vi "test Add Alias With Extra Empty Items.vi"(8 "error in (no error)":errorcluster, 11 "TestCase in":refnum<class "Routing and Faulting Aliases Unit Tests.lvclass">) -> (0 "error out":errorcluster, 3 "TestCase out":refnum<class "Routing and Faulting Aliases Unit Tests.lvclass">)   [LabVIEW 2019, in "Routing and Faulting Aliases Unit Tests.lvclass"]
uses:
  Routing and Faulting Aliases Unit Tests.lvclass
  System Explorer/Alias.ctl
  System Explorer/Endpoint.ctl
  Shared/Alias Endpoint.ctl
  Shared/Alias Mapping.ctl
  Routing and Faulting Aliases Unit Tests.lvclass/Routing and Faulting Aliases Unit Tests.ctl
  <vilib>/addons/_JKI Toolkits/VI Tester/TestCase.llb/TestCase.lvclass
  System Explorer/Routing and Faulting System Explorer.lvlib
  Scripting/Routing and Faulting Scripting.lvlib
  Shared/Routing and Faulting Shared.lvlib
  C:/Program Files (x86)/National Instruments/LabVIEW 2019/vi.lib/addons/_JKI Toolkits/VI Tester/TestCase.llb/TestCase.lvclass
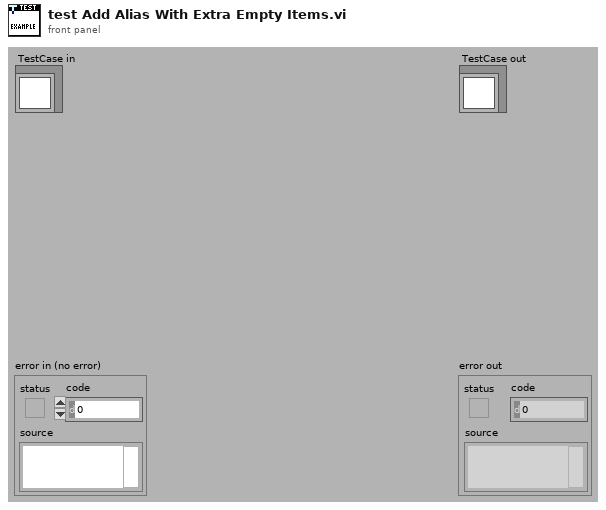
[diagram p1: front panel]
types:
  T1 = typedef "Routing and Faulting Shared.lvlib/Alias Mapping.ctl" = cluster{"Alias":string, "Endpoint":T2}
  T2 = typedef "Routing and Faulting Shared.lvlib/Alias Endpoint.ctl" = cluster{"Module Path":string, "Endpoint":string}
  T3 = typedef "Routing and Faulting System Explorer.lvlib/Endpoint.ctl" = string
  T4 = typedef "Routing and Faulting System Explorer.lvlib/Alias.ctl" = cluster{"Endpoint":T3, "Alias":string, "Remove":bool}
  T5 = typedef "Custom Device API.lvlib/Custom Device Item Ref.ctl" = u64
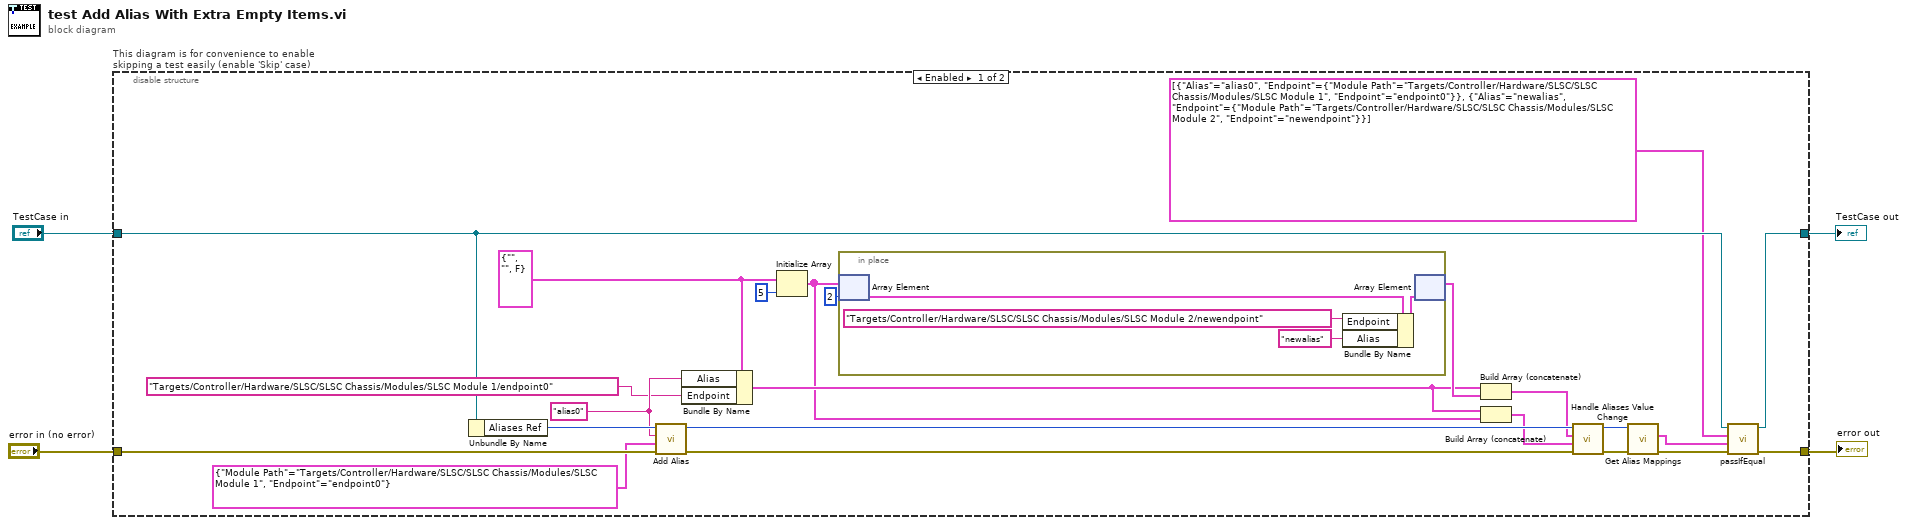
[diagram p0: block diagram]
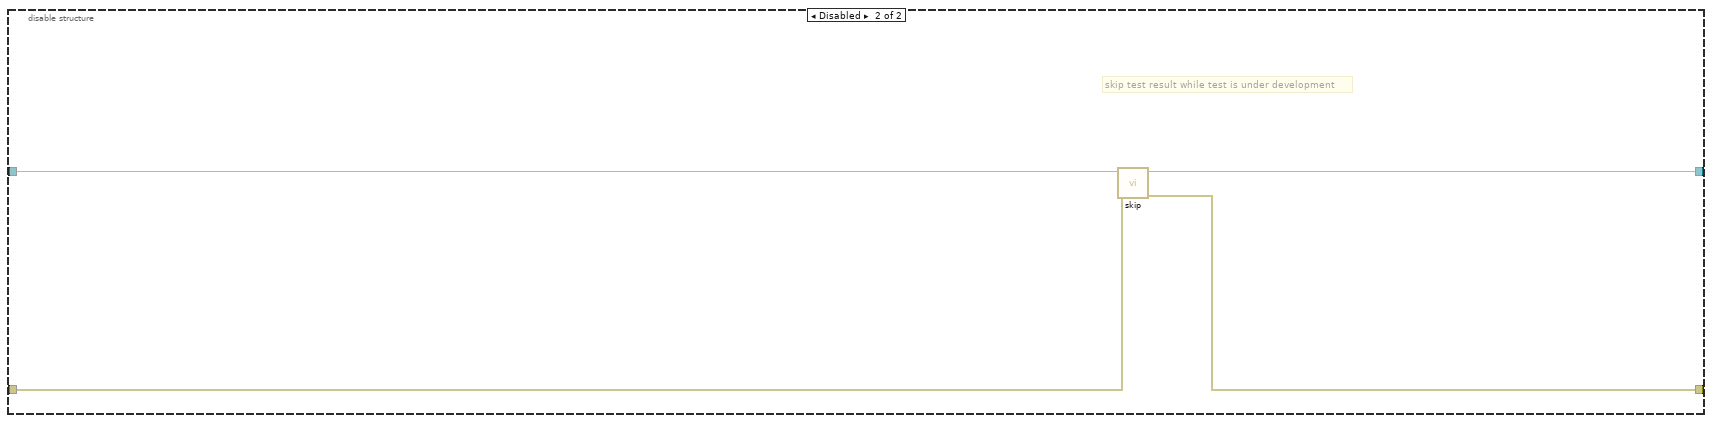
[diagram p2: hidden frame]
diagram:
  n1 = disable-structure "This diagram is for convenience to enable skipping a test easily (enable 'Skip' case)" shown="Enabled" {
    disable-tunnel: "TestCase in" -> [w22 w35]
    disable-tunnel: [w21 w33] -> w1
    disable-tunnel: [w24 w34] -> w3
    disable-tunnel: "error in (no error)" -> [w19 w32]
    frame Enabled {
      w14 = T4 {"Endpoint"="", "Alias"="", "Remove"=FALSE} ("Alias")
      w13 = "alias0" ("Alias")
      n2 = Unbundle By Name(w22) -> ("Aliases Ref"=w20:T5)
      n3 = call "Add Alias.vi"("error in"=w19, "endpoint"=T2 {"Module Path"="Targets/Controller/Hardware/SLSC/SLSC Chassis/Modules/SLSC Module 1", "Endpoint"="endpoint0"} ("Endpoint"), "alias"=w13, "endpoint aliases in"=w20) -> ("error out"=w17:errorcluster, "endpoint aliases out"=w18:T5)  [unwired: 6 in]
      n4 = Bundle By Name(cluster=w14, "Alias"=w13, "Endpoint"=T3 "Targets/Controller/Hardware/SLSC/SLSC Chassis/Modules/SLSC Module 1/endpoint0") -> (w11:T4)
      n5 = Initialize Array(w14, 5 ("dimension size")) -> (w10:T4[])
      n6 = in-place {
        n7 = in-place-array #1(w10, 2) -> (w31:T4)
        n8 = Bundle By Name(cluster=w31, "Endpoint"=T3 "Targets/Controller/Hardware/SLSC/SLSC Chassis/Modules/SLSC Module 2/newendpoint", "Alias"="newalias") -> (w28:T4)
        n9 = in-place-array #1(w28) -> (w12:T4[])  [unwired: 1 out]
      }
      n10 = Build Array (concatenate)(w11, w12) -> (w8:T4[])
      n11 = Build Array (concatenate)(w11, w10) -> (w9:T4[])
      n12 = call "Handle Aliases Value Change.vi"("error in (no error)"=w17, "OldVal"=w9, "NewVal"=w8, "Aliases Ref in"=w18) -> ("error out"=w27:errorcluster, "Aliases Ref out"=w26:T5)  [unwired: 4 in, 2 out]
      n13 = call "Get Alias Mappings.vi"("error in"=w27, "endpoint aliases in"=w26) -> ("error out"=w25:errorcluster, "alias mappings"=w23:T1[])  [unwired: 7 in, 1 out]
      n14 = call-dynamic "passIfEqual.vi"("error in (no error)"=w25, "y"=w23, "x"=T1[] [{"Alias"="alias0", "Endpoint"={"Module Path"="Targets/Controller/Hardware/SLSC/SLSC Chassis/Modules/SLSC Module 1", "Endpoint"="endpoint0"}}, {"Alias"="newalias", "Endpoint"={"Module Path"="Targets/Controller/Hardware/SLSC/SLSC Chassis/Modules/SLSC Module 2", "Endpoint"="newendpoint"}}] ("Alias Mappings"), "TestCase in"=w22) -> ("error out"=w24:errorcluster, "TestCase out"=w21:refnum<class "Routing and Faulting Aliases Unit Tests.lvclass">)  [unwired: 6 in]
    }
    frame Disabled {
      # "skip test result while test is under development"
      n15 = call <vilib>:"skip.vi"("error in (no error)"=w32, "TestCase in"=w35) -> ("error out"=w34:errorcluster, "TestCase out"=w33:refnum<class "Routing and Faulting Aliases Unit Tests.lvclass">)  [unwired: 8 in]
    }
  }
  "error out" <- w3
  "TestCase out" <- w1
